vi "Write Pull.vi"(7 "GPIO":refnum<class "GPIO.lvclass">, 8 "error in (no error)":errorcluster, 10 "GPIO Pull":T1, 11 "Session In":refnum<class "Session.lvclass">) -> (0 "error out":errorcluster, 3 "Session Out":refnum<class "Session.lvclass">)   [LabVIEW 2020, in "CTI.lvlib" / "GPIO.lvclass"]
uses:
  GPIO.lvclass
  Session/Session.lvclass
  GPIO Pull.ctl
  CTI.lvlib
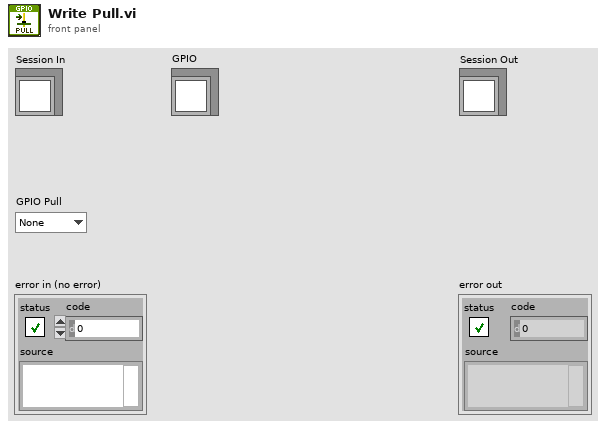
[diagram p1: front panel]
types:
  T1 = typedef "CTI.lvlib/GPIO Pull.ctl" = enum16{"None", "Up", "Down", "Both"}
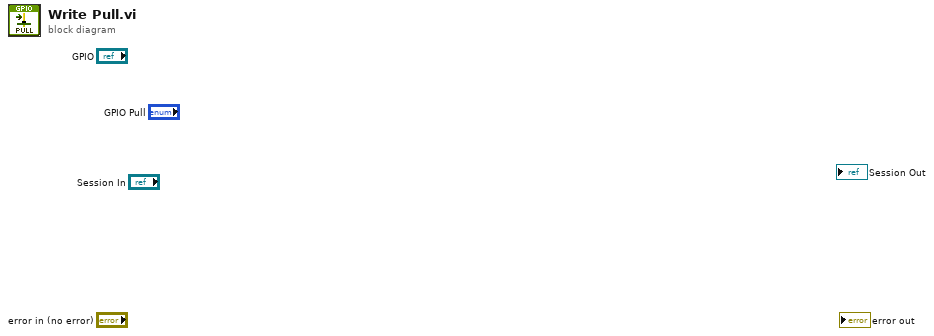
[diagram p0: block diagram]
diagram:
